vi "0-Draw Waypoints.vi"(0 "Image In":T5, 1 "Current Waypoint #":T1=-1, 2 "Waypoints List":T2, 3 "Image Descriptor":T3={"Upper-Left Corner Coordinates"={"UTM Zone"=0.0, "Hemisphere"=enum."North", "East"=0.0, "North"=0.0}, "Meters/Pixel"=42.294203} {"Upper-Left Corner Coordinates"."North" format="%#_10f"; "Upper-Left Corner Coordinates"."East" format="%#_8f"}, 4 "Font Size":i16) -> (5 "Image Out":T5, 6 "Coordinate Outside Image":bool)   [LabVIEW 2011]
doc: "Overlays waypoints onto the map image. Also includes a single 'shifted waypoint' with its own color."
uses:
  <vilib>/vision/Image Controls.llb/IMAQ Image.ctl
  0-Image Descriptor.ctl
  2-Think/2 Typedefs/UTM Location.ctl
  0x2-OCU-Think Comm/0x2 Typedefs/Waypoints List.ctl
  2-Think/2 Classes/Waypoint/Waypoint.lvclass
  0x2-OCU-Think Comm/0x2 Typedefs/Current Waypoint.ctl
  2-Think/2 Globals/2 Global.vi
panel:
  in  "number of waypts to show":i32=8
  in  "Shifted Waypt Color":u32(colorbox)=16776704
  in  "Current Waypt Color":u32(colorbox)=2815743
  in  "Finished Waypt Color":u32(colorbox)=65295
  in  "Waypt Color":u32(colorbox)=16711680
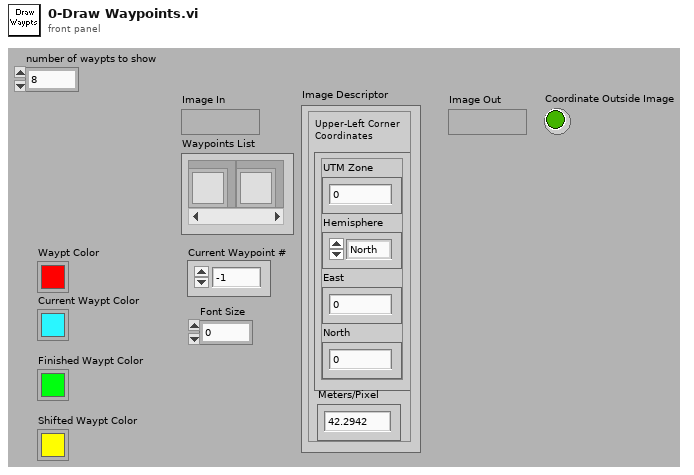
[diagram p1: front panel]
types:
  T1 = typedef "Current Waypoint.ctl" = i32
  T2 = typedef "Waypoints List.ctl" = refnum<class "Waypoint.lvclass">[]
  T3 = typedef "0-Image Descriptor.ctl" = cluster{"Upper-Left Corner Coordinates":T4, "Meters/Pixel":dbl}
  T4 = typedef "UTM Location.ctl" = cluster{"UTM Zone":dbl, "Hemisphere":enum16{"North", "South"}, "East":dbl, "North":dbl}
  T5 = typedef "IMAQ Image.ctl" = refnum<image>
  T6 = cluster{"Desired Font (Application)":enum16{"User-specified Font", "Application Font", "System Font", "Dialog Font"}, "[User-specified Font]":cluster{"Font Name":string, "Size":i16, "Strikeout?":bool, "Italic?":bool, "Underline?":bool, "Outline?":bool, "Shadow?":bool, "Bold?":bool, "Rotation Angle":dbl}, "Horizontal Alignment":i16, "Vertical Alignment":i16}
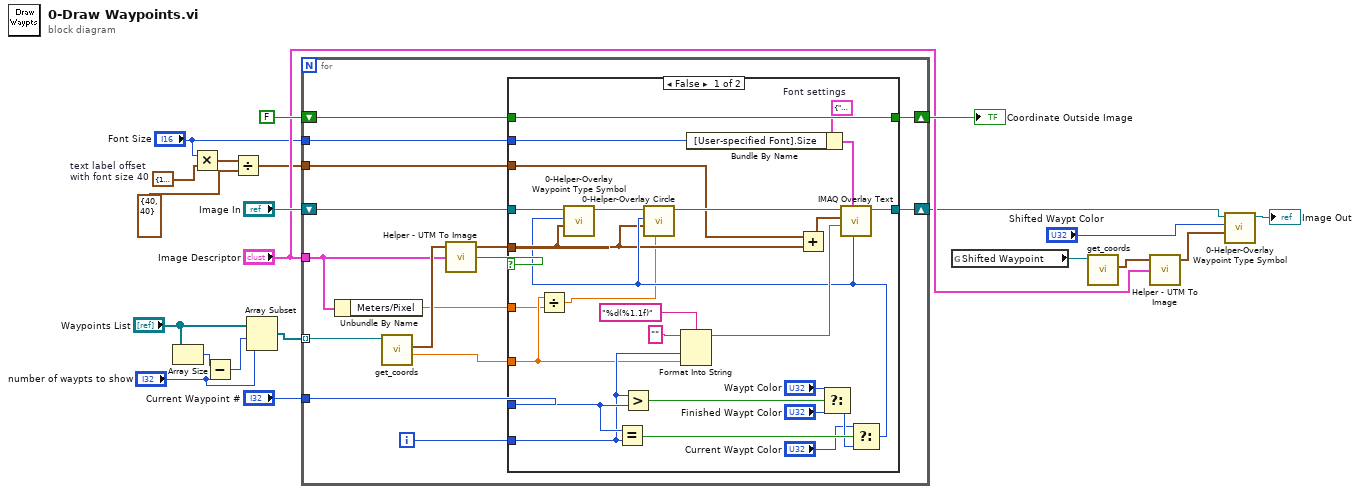
[diagram p0: block diagram]
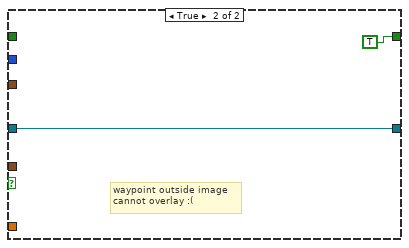
[diagram p2: hidden frame]
diagram:
  w9 = cluster{"X":i32, "Y":i32} {"X"=10, "Y"=21}  # text label offset with font size 40
  n1 = Array Size(array="Waypoints List") -> (size(s)=w3:i32)
  n2 = Multiply(x="Font Size", y=w9) -> (x*y=w8:cluster{"X":i32, "Y":i32})
  n3 = Subtract(x=w3, y="number of waypts to show") -> (x-y=w2:i32)
  n4 = Divide(x=w8, y=cluster{"X":i32, "Y":i32} {"X"=40, "Y"=40}) -> (x/y=w6:cluster{"X":dbl, "Y":dbl})
  n5 = Array Subset(array="Waypoints List", index=w2, length="number of waypts to show") -> (w5:T2)
  n6 = for {
    tunnel: w5 -> [w26] mode=indexing
    shift-right: [w35] -> w12
    shift-left: "Image In" -> [w36]
    tunnel: "Image Descriptor" -> [w25]
    tunnel: "Current Waypoint #" -> [w34]
    shift-right: [w31] -> w19
    shift-left: FALSE -> [w30]
    tunnel: "Font Size" -> [w23]
    tunnel: w6 -> [w22]
    i -> [w29]
    n7 = Unbundle By Name(w25) -> ("Meters/Pixel"=w24:dbl)
    n8 = call-dynamic "get_coords.vi"("Waypoint in"=w26) -> ("Tolerance (meters?)"=w27:dbl, "Coords"=w28:T4)  [unwired: 7 in, 2 out]
    n9 = call "Helper - UTM To Image.vi"("Image Descriptor"=w25, "UTM Location"=w28) -> ("Coordinate Outside Image"=w32:bool, "Pixel Coordinates"=w33:cluster{"X":i32, "Y":i32})  [unwired: 1 in, 1 out]
    n10 = case shown="False" w32 {
      tunnel: w36 -> [w50 w64]
      tunnel: [w61 w64] -> w35
      tunnel: w27 -> [w43 _]
      tunnel: w34 -> [w56 _]
      tunnel: w33 -> [w44 _]
      tunnel: [w51 TRUE] -> w31
      tunnel: w30 -> [w51 _]
      tunnel: w29 -> [w48 _]
      tunnel: w24 -> [w42 _]
      tunnel: w23 -> [w38 _]
      tunnel: w22 -> [w37 _]
      frame False {
        w40 = T6 {"Desired Font (Application)"=enum."User-specified Font", "[User-specified Font]"={"Font Name"="Arial Unicode MS", "Size"=40, "Strikeout?"=FALSE, "Italic?"=FALSE, "Underline?"=FALSE, "Outline?"=FALSE, "Shadow?"=FALSE, "Bold?"=TRUE, "Rotation Angle"=0.0}, "Horizontal Alignment"=0, "Vertical Alignment"=0}  # Font settings
        n11 = Divide(x=w43, y=w42) -> (x/y=w41:dbl)
        n12 = Equal?(x=w56, y=w48) -> (x = y?=w55:bool)
        n13 = Greater?(x=w48, y=w56) -> (0:w59:bool)
        n14 = Format Into String(format string="%d(%1.1f)", initial string="", w48, w43) -> (resulting string=w52:string)  [unwired: 1 in, 1 out]
        n15 = Bundle By Name(cluster=w40, "[User-specified Font].Size"=w38) -> (w39:T6)
        n16 = Add(x=w37, y=w44) -> (x+y=w62:cluster{"X":dbl, "Y":dbl})
        n17 = Select(t="Waypt Color", s=w59, f="Finished Waypt Color") -> (s? t:f=w54:u32)
        n18 = Select(t="Current Waypt Color", s=w55, f=w54) -> (s? t:f=w45:u32)
        n19 = call "0-Helper-Overlay Waypoint Type Symbol.vi"("Overlay Location"=w44, "Icon Color"=w45, "Image in"=w50) -> ("Image out"=w47:T5)  [unwired: 7 in, 1 out]
        n20 = call "0-Helper-Overlay Circle.vi"("Radius (px)"=w41, "Pixel Coordinates"=w44, "Color"=w45, "Image in"=w47) -> ("Image out"=w46:T5)  [unwired: 7 in]
        n21 = call "IMAQ Overlay Text"("Text Color (black)"=w45, "Font, Size & Style"=w39, "String"=w52, "Origin"=w62, "Image"=w46) -> ("Image Out"=w61:T5)  [unwired: 3 in, 3 out]
      }
      frame True {
        # "waypoint outside image\ncannot overlay :("
      }
    }
  }
  "Coordinate Outside Image" <- w19
  n22 = global read "2 Global.vi" "Shifted Waypoint"() -> (w16:refnum<class "Waypoint.lvclass">)
  n23 = call-dynamic "get_coords.vi"("Waypoint in"=w16) -> ("Coords"=w15:T4)  [unwired: 7 in, 3 out]
  n24 = call "Helper - UTM To Image.vi"("Image Descriptor"="Image Descriptor", "UTM Location"=w15) -> ("Pixel Coordinates"=w13:cluster{"X":i32, "Y":i32})  [unwired: 1 in, 2 out]
  n25 = call "0-Helper-Overlay Waypoint Type Symbol.vi"("Overlay Location"=w13, "Icon Color"="Shifted Waypt Color", "Image in"=w12) -> ("Image out"=→"Image Out":T5)  [unwired: 7 in, 1 out]
